vi "20211225 main.vi"() -> ()   [LabVIEW 2019]
uses:
  subVI/move/position cluster.ctl
  subVI/move/move array.ctl
  subVI/arduino/Servo/servo option.ctl
panel:
  in  "error in (no error)":errorcluster
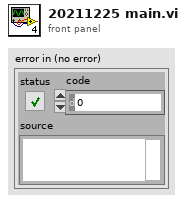
[diagram p1: front panel]
types:
  T1 = typedef "servo option.ctl" = enum8{"", "put", "catch", "vision-1", "vision-2"}
  T2 = typedef "move array.ctl" = cluster{"X":dbl, "Y":dbl}[]
  T3 = typedef "position cluster.ctl" = cluster{"X":dbl, "Y":dbl, "Angle":dbl}
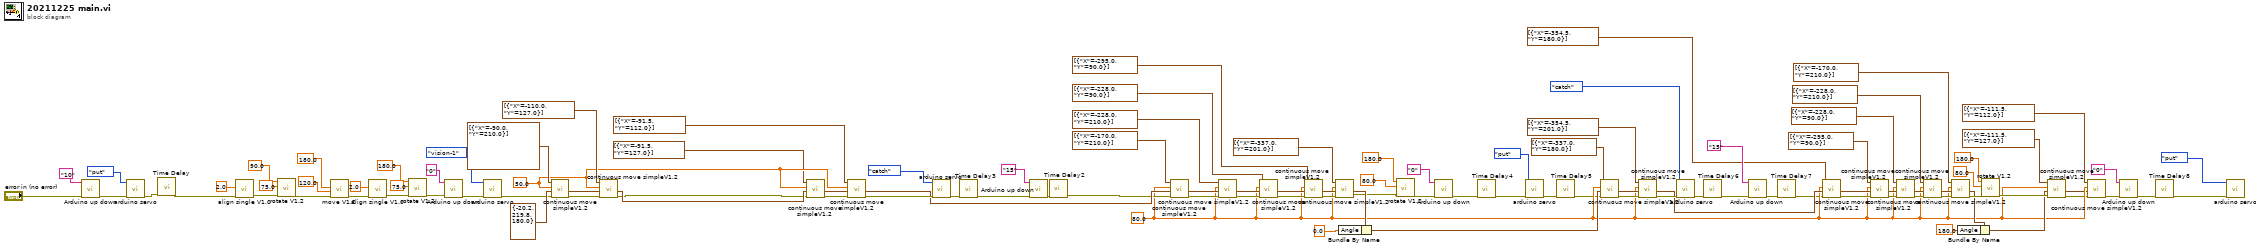
[diagram p0: block diagram]
diagram:
  w14 = 80.0 ("Speed")
  w85 = 50.0 ("Speed")
  n1 = call "Arduino up down.vi"("error in (no error)"="error in (no error)", "Height"="10") -> ("error out"=w92:errorcluster)  [unwired: 9 in]
  n2 = call "arduino servo.vi"("error in (no error)"=w92, "Enum"=enum8{"", "put", "catch"}."put") -> ("error out"=w90:errorcluster)  [unwired: 9 in]
  n3 = call "Time Delay"("error in (no error)"=w90) -> ("error out"=w89:errorcluster)  [unwired: 10 in]
  n4 = call "align single V1.0.vi"("error in (no error)"=w89, "Target (Volt)"=2.0) -> ("error out"=w110:errorcluster)  [unwired: 9 in]
  n5 = call "rotate V1.2.vi"("error in (no error)"=w110, "speed"=75.0, "degree"=90.0) -> ("error out"=w107:errorcluster)  [unwired: 8 in]
  n6 = call "move V1.2.vi"("error in (no error)"=w107, "RPM"=120.0, "Y"=180.0) -> ("error out"=w103:errorcluster)  [unwired: 8 in]
  n7 = call "align single V1.0.vi"("error in (no error)"=w103, "Target (Volt)"=2.0) -> ("error out"=w97:errorcluster)  [unwired: 9 in]
  n8 = call "rotate V1.2.vi"("error in (no error)"=w97, "speed"=75.0, "degree"=180.0) -> ("error out"=w95:errorcluster)  [unwired: 8 in]
  n9 = call "Arduino up down.vi"("error in (no error)"=w95, "Height"="0") -> ("error out"=w68:errorcluster)  [unwired: 9 in]
  n10 = call "arduino servo.vi"("error in (no error)"=w68, "Enum"=servo_option."vision-1") -> ("error out"=w69:errorcluster)  [unwired: 9 in]
  n11 = call "continuous move simpleV1.2.vi"("error in (no error)"=w69, "Position"=T3 {"X"=-20.2, "Y"=219.8, "Angle"=180.0}, "Speed"=w85, "Array"=T2 [{"X"=-90.0, "Y"=210.0}]) -> ("error out"=w94:errorcluster, "Position out"=w93:T3)  [unwired: 6 in]
  n12 = call "continuous move simpleV1.2.vi"("error in (no error)"=w94, "Position"=w93, "Speed"=w85, "Array"=T2 [{"X"=-110.0, "Y"=127.0}]) -> ("error out"=w26:errorcluster, "Position out"=w86:T3)  [unwired: 6 in]
  n13 = call "continuous move simpleV1.2.vi"("error in (no error)"=w26, "Position"=w86, "Speed"=w85, "Array"=T2 [{"X"=-91.5, "Y"=127.0}]) -> ("error out"=w83:errorcluster, "Position out"=w84:T3)  [unwired: 6 in]
  n14 = call "continuous move simpleV1.2.vi"("error in (no error)"=w83, "Position"=w84, "Speed"=w85, "Array"=T2 [{"X"=-91.5, "Y"=112.0}]) -> ("error out"=w82:errorcluster, "Position out"=w79:T3)  [unwired: 6 in]
  n15 = call "arduino servo.vi"("error in (no error)"=w82, "Enum"=servo_option."catch") -> ("error out"=w59:errorcluster)  [unwired: 9 in]
  n16 = call "Time Delay3"("error in (no error)"=w59) -> ("error out"=w60:errorcluster)  [unwired: 10 in]
  n17 = call "Arduino up down.vi"("error in (no error)"=w60, "Height"="15") -> ("error out"=w71:errorcluster)  [unwired: 9 in]
  n18 = call "Time Delay2"("error in (no error)"=w71) -> ("error out"=w70:errorcluster)  [unwired: 10 in]
  n19 = call "continuous move simpleV1.2.vi"("error in (no error)"=w70, "Position"=w79, "Speed"=w14, "Array"=T2 [{"X"=-170.0, "Y"=210.0}]) -> ("error out"=w75:errorcluster, "Position out"=w76:T3)  [unwired: 6 in]
  n20 = call "continuous move simpleV1.2.vi"("error in (no error)"=w75, "Position"=w76, "Speed"=w14, "Array"=T2 [{"X"=-228.0, "Y"=210.0}]) -> ("error out"=w72:errorcluster, "Position out"=w73:T3)  [unwired: 6 in]
  n21 = call "continuous move simpleV1.2.vi"("error in (no error)"=w72, "Position"=w73, "Speed"=w14, "Array"=T2 [{"X"=-228.0, "Y"=90.0}]) -> ("error out"=w66:errorcluster, "Position out"=w65:T3)  [unwired: 6 in]
  n22 = call "continuous move simpleV1.2.vi"("error in (no error)"=w66, "Position"=w65, "Speed"=w14, "Array"=T2 [{"X"=-295.0, "Y"=90.0}]) -> ("error out"=w63:errorcluster, "Position out"=w62:T3)  [unwired: 6 in]
  n23 = call "continuous move simpleV1.2.vi"("error in (no error)"=w63, "Position"=w62, "Speed"=w14, "Array"=T2 [{"X"=-337.0, "Y"=201.0}]) -> ("error out"=w56:errorcluster, "Position out"=w58:T3)  [unwired: 6 in]
  n24 = Bundle By Name(cluster=w58, "Angle"=0.0 ("X")) -> (w48:T3)
  n25 = call "rotate V1.2.vi"("error in (no error)"=w56, "speed"=80.0 ("RPM"), "degree"=180.0 ("Y")) -> ("error out"=w52:errorcluster)  [unwired: 8 in]
  n26 = call "Arduino up down.vi"("error in (no error)"=w52, "Height"="0") -> ("error out"=w51:errorcluster)  [unwired: 9 in]
  n27 = call "Time Delay4"("error in (no error)"=w51) -> ("error out"=w50:errorcluster)  [unwired: 10 in]
  n28 = call "arduino servo.vi"("error in (no error)"=w50, "Enum"=servo_option."put") -> ("error out"=w8:errorcluster)  [unwired: 9 in]
  n29 = call "Time Delay5"("error in (no error)"=w8) -> ("error out"=w9:errorcluster)  [unwired: 10 in]
  n30 = call "continuous move simpleV1.2.vi"("error in (no error)"=w9, "Position"=w48, "Speed"=w14, "Array"=T2 [{"X"=-337.0, "Y"=180.0}]) -> ("error out"=w46:errorcluster, "Position out"=w45:T3)  [unwired: 6 in]
  n31 = call "continuous move simpleV1.2.vi"("error in (no error)"=w46, "Position"=w45, "Speed"=w14, "Array"=T2 [{"X"=-354.5, "Y"=201.0}]) -> ("error out"=w42:errorcluster, "Position out"=w40:T3)  [unwired: 6 in]
  n32 = call "arduino servo.vi"("error in (no error)"=w42, "Enum"=servo_option."catch") -> ("error out"=w7:errorcluster)  [unwired: 9 in]
  n33 = call "Time Delay6"("error in (no error)"=w7) -> ("error out"=w6:errorcluster)  [unwired: 10 in]
  n34 = call "Arduino up down.vi"("error in (no error)"=w6, "Height"="15") -> ("error out"=w4:errorcluster)  [unwired: 9 in]
  n35 = call "Time Delay7"("error in (no error)"=w4) -> ("error out"=w5:errorcluster)  [unwired: 10 in]
  n36 = call "continuous move simpleV1.2.vi"("error in (no error)"=w5, "Position"=w40, "Speed"=w14, "Array"=T2 [{"X"=-354.5, "Y"=180.0}]) -> ("error out"=w38:errorcluster, "Position out"=w36:T3)  [unwired: 6 in]
  n37 = call "continuous move simpleV1.2.vi"("error in (no error)"=w38, "Position"=w36, "Speed"=w14, "Array"=T2 [{"X"=-295.0, "Y"=90.0}]) -> ("error out"=w35:errorcluster, "Position out"=w34:T3)  [unwired: 6 in]
  n38 = call "continuous move simpleV1.2.vi"("error in (no error)"=w35, "Position"=w34, "Speed"=w14, "Array"=T2 [{"X"=-228.0, "Y"=90.0}]) -> ("error out"=w33:errorcluster, "Position out"=w32:T3)  [unwired: 6 in]
  n39 = call "continuous move simpleV1.2.vi"("error in (no error)"=w33, "Position"=w32, "Speed"=w14, "Array"=T2 [{"X"=-228.0, "Y"=210.0}]) -> ("error out"=w29:errorcluster, "Position out"=w28:T3)  [unwired: 6 in]
  n40 = call "continuous move simpleV1.2.vi"("error in (no error)"=w29, "Position"=w28, "Speed"=w14, "Array"=T2 [{"X"=-170.0, "Y"=210.0}]) -> ("error out"=w23:errorcluster, "Position out"=w20:T3)  [unwired: 6 in]
  n41 = Bundle By Name(cluster=w20, "Angle"=180.0) -> (w17:T3)
  n42 = call "rotate V1.2.vi"("error in (no error)"=w23, "speed"=80.0 ("RPM"), "degree"=180.0 ("Y")) -> ("error out"=w18:errorcluster)  [unwired: 8 in]
  n43 = call "continuous move simpleV1.2.vi"("error in (no error)"=w18, "Position"=w17, "Speed"=w14, "Array"=T2 [{"X"=-111.5, "Y"=127.0}]) -> ("error out"=w12:errorcluster, "Position out"=w13:T3)  [unwired: 6 in]
  n44 = call "continuous move simpleV1.2.vi"("error in (no error)"=w12, "Position"=w13, "Speed"=w14, "Array"=T2 [{"X"=-111.5, "Y"=112.0}]) -> ("error out"=w11:errorcluster)  [unwired: 6 in, 1 out]
  n45 = call "Arduino up down.vi"("error in (no error)"=w11, "Height"="0") -> ("error out"=w3:errorcluster)  [unwired: 9 in]
  n46 = call "Time Delay8"("error in (no error)"=w3) -> ("error out"=w2:errorcluster)  [unwired: 10 in]
  n47 = call "arduino servo.vi"("error in (no error)"=w2, "Enum"=servo_option."put") -> ()  [unwired: 9 in, 1 out]
